vi "AlicatTester.vi"() -> ()   [LabVIEW 2020]
uses:
  7500c3e5-3861-b947-859a-5441f3d08f62.vi
panel:
  in  "RestekPort":refnum<visa-resource-name>="ASRL3::INSTR"
  in  "AlicatIP":string="10.245.24.4"
  in  "Stop":bool
  in  "settling(ms)":u32=500
  out "values":dbl[][](array[numeric])
  in  "SPinc":dbl=0.0005
  out "XY Graph":cluster{dbl[], dbl[]}(graph)
  in  "SPstop":dbl=0.00785
  in  "SPstart":dbl=0.001
  in  "holdLoops":i32=5
  # "https://wiki.4winds.tools/index.php/Alicat"
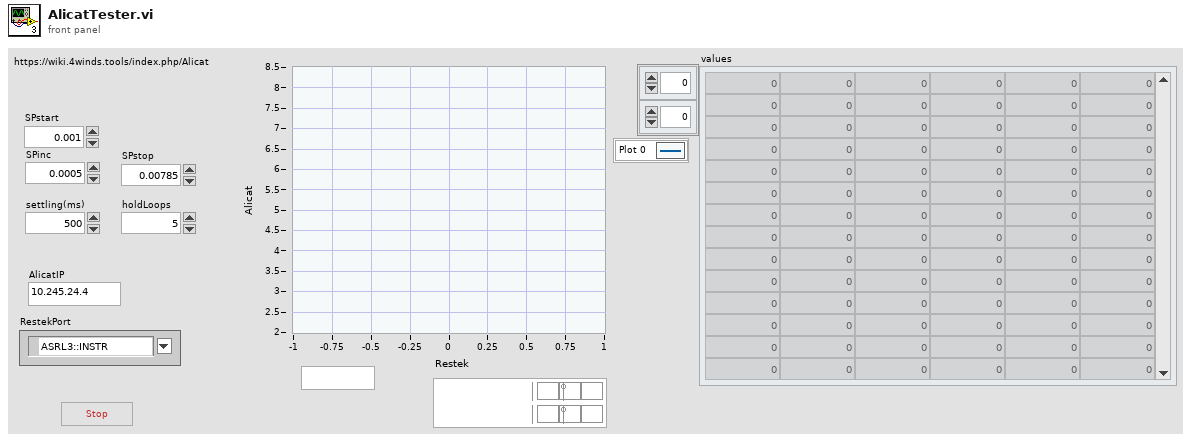
[diagram p1: front panel]
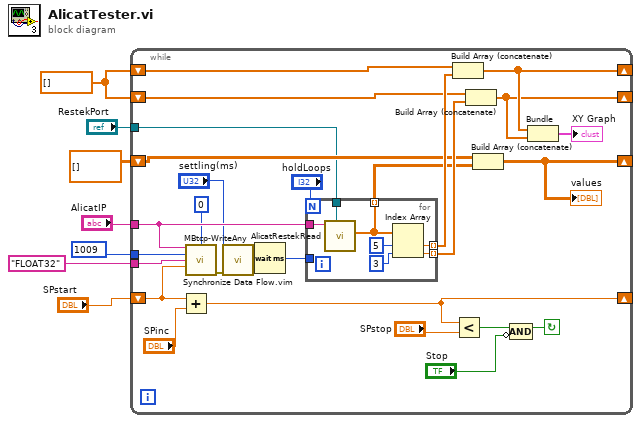
[diagram p0: block diagram]
diagram:
  w5 = dbl[] []
  n1 = while {
    tunnel: "AlicatIP" -> [w33]
    shift-right: [w31] -> _
    shift-left: "SPstart" -> [w32]
    shift-right: [w24] -> _
    shift-left: w5 -> [w27]
    shift-right: [w23] -> _
    shift-left: w5 -> [w26]
    tunnel: 1009 ("Register") -> [w20]
    tunnel: "FLOAT32" ("DataType(:RegisterType)") -> [w19]
    shift-right: [w11] -> _
    shift-left: dbl[][] [] -> [w12]
    tunnel: "RestekPort" -> [w8]
    stop <- w10 continue-if-true
    n2 = Add(x=w32, y="SPinc") -> (x+y=w31:dbl)
    n3 = call "MBtcp-WriteAny.vi"("IP Address"=w33, "Slave ID"=u8 0, "Register"=w20, "DataType(:RegisterType)"=w19, "Value to Output"=w32) -> ("error out"=w16:errorcluster)  [unwired: 10 in]
    n4 = call "Synchronize Data Flow.vim"("input 4"=w16, "input 1"="settling(ms)") -> ("output 1"=w14:u32)  [unwired: 2 in, 3 out]
    n5 = Wait (ms)(milliseconds to wait=w14) -> (millisecond timer value=w17:u32)
    n6 = for {
      N: "holdLoops" -> [_]
      tunnel: w33 -> [w41]
      tunnel: [w38] -> w28 mode=indexing
      tunnel: [w37] -> w25 mode=indexing
      tunnel: [w36] -> w13 mode=indexing
      tunnel: w17 -> [_]
      tunnel: w8 -> [w35]
      n7 = call "AlicatRestekRead.vi"("Restek ProFLOW 6000 port"=w35, "IP Address"=w41) -> ("values"=w36:dbl[])  [unwired: 9 in]
      n8 = Index Array(array=w36, index #1=5 ("index"), index #2=3 ("index")) -> (element #1=w38:dbl, element #2=w37:dbl)
    }
    n9 = Build Array (concatenate)(w27, w28) -> (w24:dbl[])
    n10 = Less?(x=w31, y="SPstop") -> (x < y?=w29:bool)
    n11 = Build Array (concatenate)(w26, w25) -> (w23:dbl[])
    n12 = Build Array (concatenate)(w12, w13) -> (w11:dbl[][])
    "values" <- w11
    n13 = Compound Arithmetic op=AND(w29, invert "Stop") -> (w10:bool)
    n14 = Bundle(w24, w23) -> (→"XY Graph":cluster{dbl[], dbl[]})  [unwired: 1 in]
  }
